vi "_builtins_rect_to_grid.vi"(10 "Grid Size (12px)":i32=12, 11 "Rects in":T1[](array[typedef])) -> (3 "Resolved Rects out":T1[](array[typedef]))   [LabVIEW 2019, in "Script.lvlib"]
doc: "Resolves the nearest grid rectangle bounds.\n\nCreated by: Ryan Pacini"
uses:
  Script.lvlib
  <vilib>/Utility/miscctls.llb/LVRectTypeDef.ctl
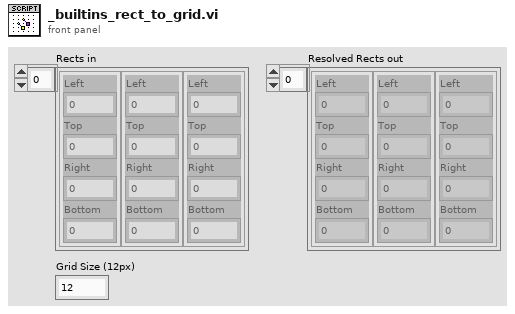
[diagram p1: front panel]
types:
  T1 = typedef "LVRectTypeDef.ctl" = cluster{"Left":i16, "Top":i16, "Right":i16, "Bottom":i16}
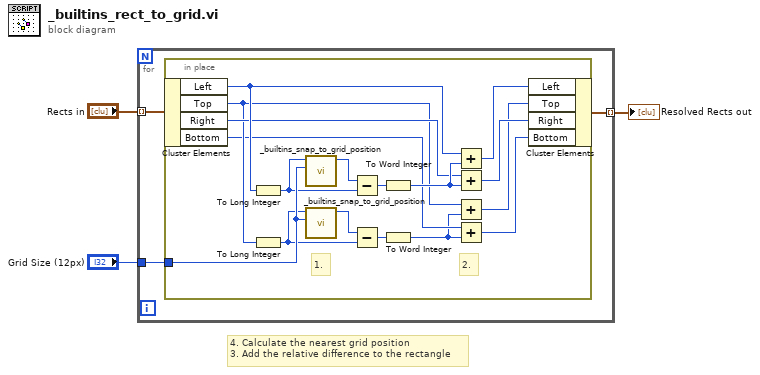
[diagram p0: block diagram]
diagram:
  # "4. Calculate the nearest grid position\n3. Add the relative difference to the rectangle"
  n1 = for {
    tunnel: "Rects in" -> [w5] mode=indexing
    tunnel: "Grid Size (12px)" -> [w6]
    tunnel: [w4] -> w1 mode=indexing
    n2 = in-place {
      in-place-border: w6 -> [w23]
      # "2."
      # "1."
      n3 = in-place-cluster #1(w5) -> ("Left"=w17:i16, "Top"=w12:i16, "Right"=w14:i16, "Bottom"=w10:i16)
      n4 = To Long Integer(number=w17) -> (32bit integer=w22:i32)
      n5 = To Long Integer(number=w12) -> (32bit integer=w19:i32)
      n6 = call "_builtins_snap_to_grid_position.vi"("Gride Size (12px)"=w23, "Abs Position"=w22) -> ("Resolved Abs Position"=w20:i32)  [unwired: 9 in]
      n7 = call "_builtins_snap_to_grid_position.vi"("Gride Size (12px)"=w23, "Abs Position"=w19) -> ("Resolved Abs Position"=w21:i32)  [unwired: 9 in]
      n8 = Subtract(x=w20, y=w22) -> (x-y=w18:i32)
      n9 = Subtract(x=w21, y=w19) -> (x-y=w8:i32)
      n10 = To Word Integer(number=w18) -> (16bit integer=w15:i16)
      n11 = To Word Integer(number=w8) -> (16bit integer=w7:i16)
      n12 = Add(x=w17, y=w15) -> (x+y=w16:i16)
      n13 = Add(x=w14, y=w15) -> (x+y=w13:i16)
      n14 = Add(x=w12, y=w7) -> (x+y=w11:i16)
      n15 = Add(x=w10, y=w7) -> (x+y=w9:i16)
      n16 = in-place-cluster #1("Left"=w16, "Top"=w11, "Right"=w13, "Bottom"=w9) -> (w4:T1)
    }
  }
  "Resolved Rects out" <- w1
